vi "Cleanup.vi"(8 "error in (no error)":errorcluster, 10 "System In":refnum<class "abs_System.lvclass">, 11 "Node in":refnum<class "abs_Type Leaf.lvclass">) -> (0 "error out":errorcluster, 2 "System Out":refnum<class "abs_System.lvclass">, 3 "Node out":refnum<class "abs_Type Leaf.lvclass">)   [LabVIEW 2021, in "BT.lvlib" / "abs_Type Leaf.lvclass"]
uses:
  abs_Type Leaf.lvclass
  abs_System/abs_System.lvclass
  abs_Type Leaf.lvclass/abs_Type Leaf.ctl
  Properties/Read Value Class.vi
  Properties/Write Value Class.vi
  LV_Abstract/Source/Abs_Types/Type/Abs_Type.lvclass
  abs_Leaf/abs_Leaf.lvclass
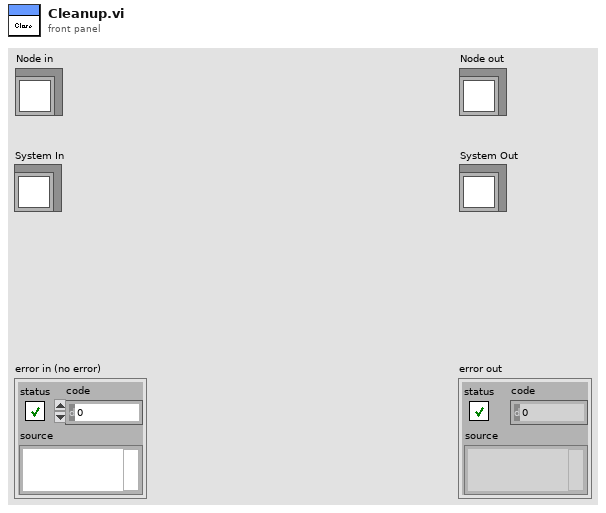
[diagram p1: front panel]
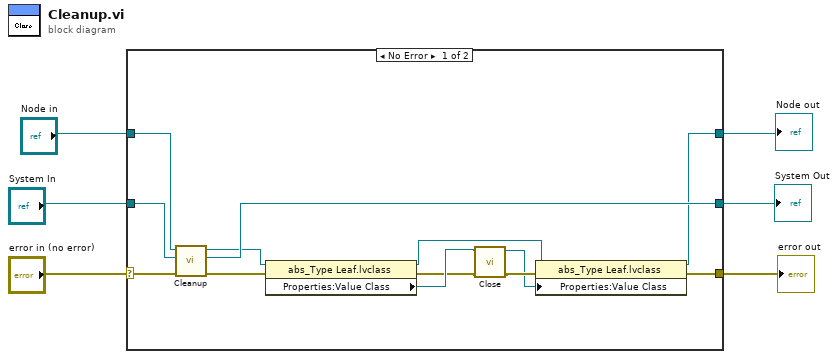
[diagram p0: block diagram]
diagram:
  n1 = case shown="No Error" "error in (no error)" {
    selector: "error in (no error)" -> [w18 w20]
    tunnel: [w19 w21] -> w5
    tunnel: "System In" -> [w17 w21]
    tunnel: "Node in" -> [w16 w22]
    tunnel: [w12 w20] -> w6
    tunnel: [w11 w22] -> w2
    frame No Error {
      n2 = call-parent "Cleanup.vi"("error in (no error)"=w18, "System In"=w17, "Node in"=w16) -> ("error out"=w15:errorcluster, "System Out"=w19:refnum<class "abs_System.lvclass">, "Node out"=w14:refnum<class "abs_Type Leaf.lvclass">)  [unwired: 6 in]
      n3 = property class="abs_Type Leaf.lvclass"(reference=w14, error in=w15) -> (reference out=w13:refnum<class "abs_Type Leaf.lvclass">, error out=w9:errorcluster, "Properties:Value Class"=w10:refnum<class "Abs_Type.lvclass">)
      n4 = call-dynamic "Close.vi"("error in (no error)"=w9, "Data in"=w10) -> ("error out"=w8:errorcluster, "Data out"=w7:refnum<class "Abs_Type.lvclass">)  [unwired: 8 in]
      n5 = property class="abs_Type Leaf.lvclass"(reference=w13, error in=w8, "Properties:Value Class"=w7) -> (reference out=w11:refnum<class "abs_Type Leaf.lvclass">, error out=w12:errorcluster)
    }
    frame Error {
    }
  }
  "error out" <- w6
  "Node out" <- w2
  "System Out" <- w5
